vi "GPack Prefs Folder.vi"(7 "Allow Creation (T)":bool=TRUE) -> (2 "error out":errorcluster, 3 "GPack Prefs Folder":path)   [LabVIEW 2020, in "GPack.lvlib" / "GPackPrefs.lvclass"]
uses:
  GPackPrefs.lvclass
  <vilib>/Utility/sysdir.llb/System Directory Type.ctl
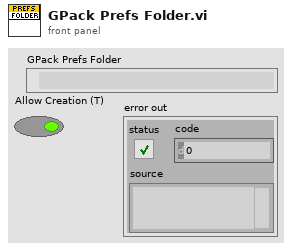
[diagram p1: front panel]
types:
  T1 = typedef "System Directory Type.ctl" = i32
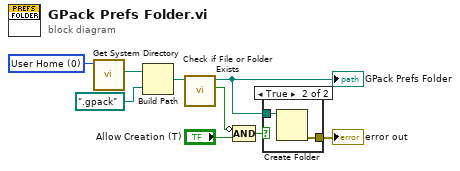
[diagram p0: block diagram]
diagram:
  w9 = T1 0 items=["User Home"=0, "User Desktop"=1, "User Documents"=2, "User Application Data"=3, "User Preferences"=4, "User Temporary"=5, "Public Documents"=6, "Public Application Data"=7, "Public Preferences"=8, "Public Cache"=13, "System Core Libraries"=9, "System Installed Libraries"=10, "Application Files"=11, "Boot Volume Root"=12] ("system directory type")
  n1 = call <vilib>:"Get System Directory.vi"("system directory type"=w9) -> ("system directory"=w8:path)  [unwired: 10 in]
  n2 = Build Path(base path=w8, name or relative path=path ".gpack") -> (appended path=w6:path)
  n3 = call <vilib>:"Check if File or Folder Exists.vi"("path"=w6) -> ("file or folder exists?"=w5:bool, "dup path"=w4:path)  [unwired: 8 in, 1 out]
  "GPack Prefs Folder" <- w4
  n4 = Compound Arithmetic op=AND(invert w5, "Allow Creation (T)") -> (w2:bool)
  n5 = case shown="True" w2 {
    tunnel: w4 -> [_ w11]
    tunnel: [_ w10] -> w3
    frame False {
    }
    frame True {
      n6 = Create Folder(path (use dialog)=w11) -> (error out=w10:errorcluster)  [unwired: 2 in, 2 out]
    }
  }
  "error out" <- w3
